vi "Fetch Trace.vi"(8 "error in (no error)":errorcluster, 9 "Timeout (10000ms)":i32=10000, 10 "Trace (1: Trace 1)":i32(ring)=1 items=["Trace 1"=1, "Trace 2"=2, "Trace 3"=3, "Trace 4"=4], 11 "VISA resource name":refnum<visa-resource-name>) -> (0 "error out":errorcluster, 2 "Trace Data":dbl[](array[numeric]), 3 "VISA resource name out":refnum<visa-resource-name>)   [LabVIEW 2022 SP3, in "Agilent N934X Series.lvlib"]
doc: "Fetches trace from the spectrum analyzer and does not initiate data acquisition.\n\nNote:\n\nThis VI does not check the instrument status. Typically, you call this VI only in a sequence of calls to other low-level instrument driver VIs. The sequence performs one operation. You use the low-level VIs to optimize one or more aspects of interaction with the instrument. If you want to check the instrument status, call the <B>Error Query VI</B> at the conclusion of the sequence."
uses:
  <instrlib>/Agilent N934X Series/Agilent N934X Series.lvlib
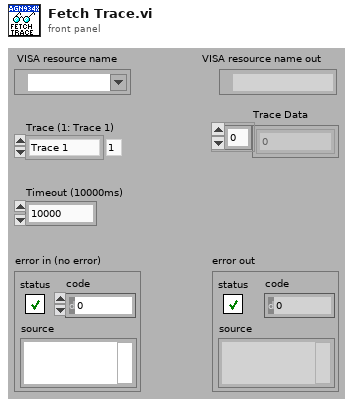
[diagram p1: front panel]
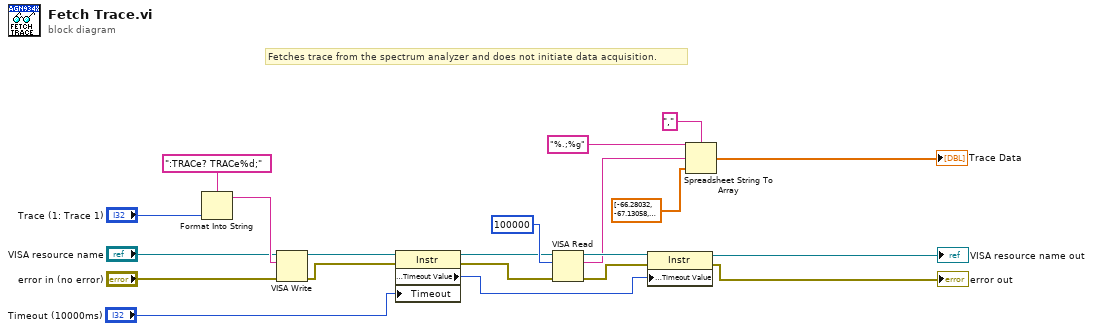
[diagram p0: block diagram]
diagram:
  # "Fetches trace from the spectrum analyzer and does not initiate data acquisition."
  n1 = Format Into String(format string=":TRACe? TRACe%d;", "Trace (1: Trace 1)") -> (resulting string=w19:string)  [unwired: 2 in, 1 out]
  n2 = VISA Write(VISA resource name="VISA resource name", write buffer=w19, error in (no error)="error in (no error)") -> (VISA resource name out=w15:refnum<visa-resource-name>, error out=w14:errorcluster)  [unwired: 1 out]
  n3 = property class="Instr"(reference=w15, error in=w14, "Timeout"="Timeout (10000ms)") -> (reference out=w13:refnum<visa-resource-name>, error out=w12:errorcluster, "General Settings:Timeout Value"=w10:u32)
  n4 = VISA Read(VISA resource name=w13, byte count=u32 100000, error in (no error)=w12) -> (VISA resource name out=w9:refnum<visa-resource-name>, read buffer=w7:string, error out=w8:errorcluster)  [unwired: 1 out]
  n5 = property class="Instr"(reference=w9, error in=w8, "General Settings:Timeout Value"=w10) -> (reference out=→"VISA resource name out":refnum<visa-resource-name>, error out=→"error out":errorcluster)
  n6 = Spreadsheet String To Array(delimiter (Tab)=",", format string="%.;%g", spreadsheet string=w7, array type (2D Dbl)=dbl[] [-66.28032, -67.13058, -67.71282, -69.11133, -72.48418, -68.59103, -74.18298, -67.65571, -67.90143, -68.77035, -69.91087, -65.28284, -72.02601, -68.77459, -70.57571] ("Trace Data")) -> (array=→"Trace Data":dbl[])
